vi "UDLR (Arrows).vi"() -> (3 "UDLR (Arrows)":string[](array[string]))   [LabVIEW 2025, in "AOC.lvlib"]
uses:
  AOC.lvlib
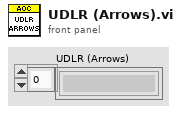
[diagram p1: front panel]
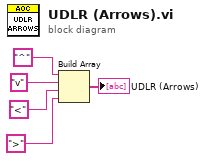
[diagram p0: block diagram]
diagram:
  n1 = Build Array("^", "v", "<", ">") -> (→"UDLR (Arrows)":string[])
